vi "加载一个资料夹内的所有图片.vi"(0 "path":path) -> (3 "subarray":string[](array[string]), 4 "该资料夹内所有图片Array":path[](array[path]))   [LabVIEW 2014]
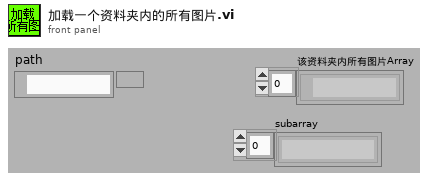
[diagram p1: front panel]
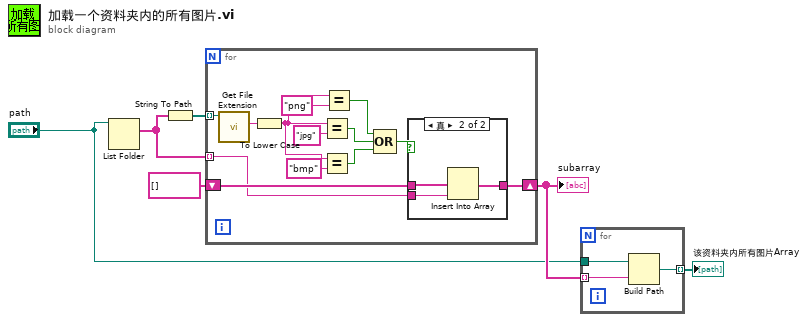
[diagram p0: block diagram]
diagram:
  n1 = List Folder(path="path") -> (filenames=w4:string[])  [unwired: 1 in, 5 out]
  n2 = String To Path(string=w4) -> (path=w5:path[])
  n3 = for {
    tunnel: w5 -> [w19] mode=indexing
    shift-right: [w11] -> w3
    shift-left: string[] [] ("subarray") -> [w12]
    tunnel: w4 -> [w10] mode=indexing
    n4 = call <vilib>:"Get File Extension.vi"("file"=w19) -> ("lowercase file extension"=w18:string)  [unwired: 1 in, 9 out]
    n5 = To Lower Case(string=w18) -> (all lower case string=w9:string)
    n6 = Equal?(x=w9, y="jpg") -> (x = y?=w15:bool)
    n7 = Equal?(x=w9, y="bmp") -> (x = y?=w14:bool)
    n8 = Equal?(x=w9, y="png") -> (x = y?=w8:bool)
    n9 = Compound Arithmetic op=OR(w8, w15, w14) -> (w13:bool)
    n10 = case shown="真" w13 {
      tunnel: w12 -> [w20 w23]
      tunnel: [w20 w21] -> w11
      tunnel: w10 -> [_ w22]
      frame False {
      }
      frame True {
        n11 = Insert Into Array(array=w23, new element=w22) -> (w21:string[])  [unwired: 1 in]
      }
    }
  }
  "subarray" <- w3
  n12 = for {
    tunnel: w3 -> [w25] mode=indexing
    tunnel: "path" -> [w26]
    tunnel: [w24] -> w2 mode=indexing
    n13 = Build Path(base path=w26, name or relative path=w25) -> (appended path=w24:path)
  }
  "该资料夹内所有图片Array" <- w2
